vi "Send Message.vi"(8 "error in (no error)":errorcluster, 10 "Path":path, 11 "Stream in":refnum<class "Stream.lvclass">) -> (0 "error out":errorcluster, 3 "Stream out":refnum<class "Stream.lvclass">)   [LabVIEW 2023, in "Stream.lvclass"]
uses:
  Stream.lvclass
  Controls/Queue Operation.ctl
  Stream.lvclass/Stream.ctl
  Message Data/Message Data.lvclass
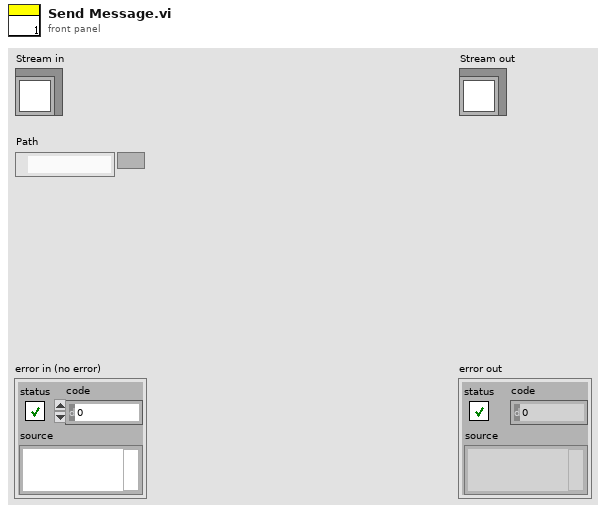
[diagram p1: front panel]
types:
  T1 = typedef "Queue Operation.ctl" = enum16{"Create & Enqueue N", "Enqueue N", "Dequeue", "Enstack N", "Flush", "Release"}
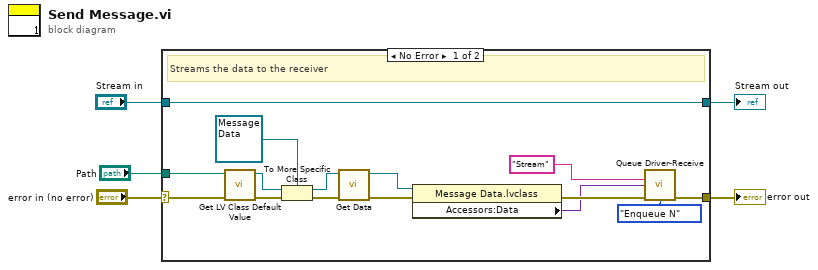
[diagram p0: block diagram]
diagram:
  n1 = case shown="No Error" "error in (no error)" {
    selector: "error in (no error)" -> [w9 w22]
    tunnel: [w16 w22] -> w4
    tunnel: [w20 w21] -> w2
    tunnel: "Stream in" -> [w20 w21]
    tunnel: "Path" -> [w8 _]
    frame No Error {
      # "Streams the data to the receiver"
      n2 = call <vilib>:"Get LV Class Default Value.vi"("error in (no error)"=w9, "class path"=w8) -> ("error out"=w14:errorcluster, "object"=w12:refnum<class>)  [unwired: 8 in]
      n3 = To More Specific Class(target class=refnum<class "Message Data.lvclass"> refnum ("Message Data.lvclass"), reference=w12, error in=w14) -> (specific class reference=w10:refnum<class "Message Data.lvclass">, error out=w13:errorcluster)
      n4 = call-dynamic "Get Data.vi"("error in (no error)"=w13, "Message Data in"=w10) -> ("error out"=w7:errorcluster, "Message Data out"=w6:refnum<class "Message Data.lvclass">)  [unwired: 8 in]
      n5 = property class="Message Data.lvclass"(reference=w6, error in=w7) -> (error out=w19:errorcluster, "Accessors:Data"=w18:variant)  [unwired: 1 out]
      n6 = call "Queue Driver-Receive.vi"("State"="Stream" ("Event Name"), "Data"=w18, "Error In"=w19, "Queue Operation"=Queue_Operation."Enqueue N") -> ("Error Out"=w16:errorcluster)  [unwired: 10 in, 1 out]
    }
    frame Error {
    }
  }
  "error out" <- w4
  "Stream out" <- w2
